vi "sd histogram.vi"() -> ()   [LabVIEW 2020]
uses:
  <vilib>/measure/NI_MABase.lvlib
panel:
  out "Waveform Graph":waveform(dbl)(graph)
  out "Gyakoriság hisztogram":T1(graph)
  out "Empirikus sûrûségfüggvény":cluster{"X Values":dbl[], dbl[]}(graph)
  out "Középérték [g]":dbl
  out "Szórás [g]":dbl
  out "Konfidencia intervallum [g]":dbl
  out "Százalékos hiba [%]":dbl
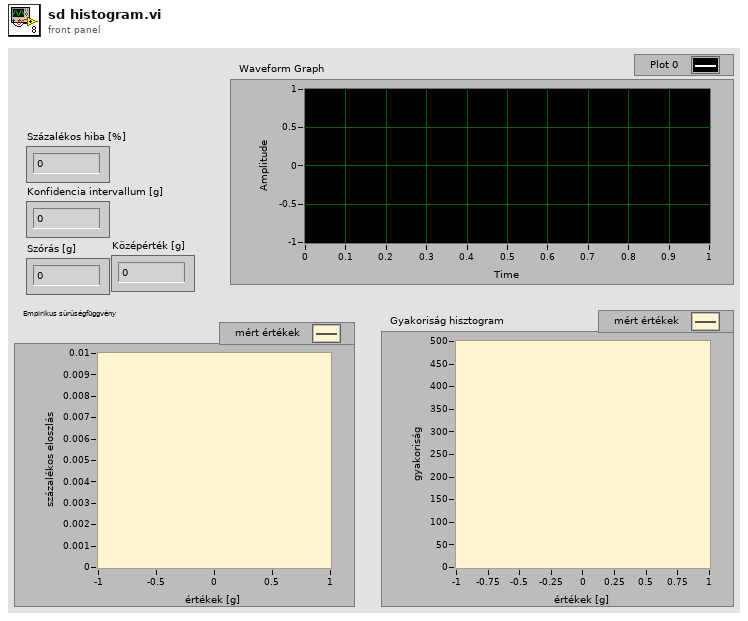
[diagram p1: front panel]
types:
  T1 = cluster{"X Values":dbl[], "Histogram: h(x)":i32[]}
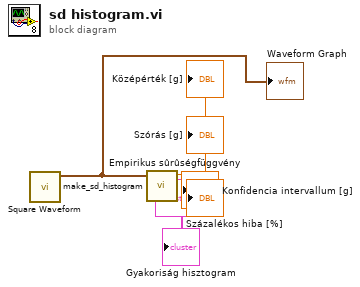
[diagram p0: block diagram]
diagram:
  n1 = call <vilib>:"Square Waveform.vi"() -> ("signal out"=w1:waveform(dbl))  [unwired: 10 in, 1 out]
  "Waveform Graph" <- w1
  n2 = call "make_sd_histogram.vi"("waveform"=w1) -> ("Százalékos hiba [%]"=→"Százalékos hiba [%]":dbl, "Konfidencia intervallum [g]"=→"Konfidencia intervallum [g]":dbl, "Szórás [g]"=→"Szórás [g]":dbl, "Középérték [g]"=→"Középérték [g]":dbl, "Empirikus sûrûségfüggvény"=→"Empirikus sûrûségfüggvény":cluster{"X Values":dbl[], dbl[]}, "Gyakoriság hisztogram"=→"Gyakoriság hisztogram":T1)  [unwired: 4 in, 1 out]
